vi "Util_ApproxEquals.vi"(8 "Tolerance":dbl=1e-09, 10 "Value 2":dbl, 11 "Value 1":dbl) -> (3 "ApproxEquals":bool)   [LabVIEW 2019]
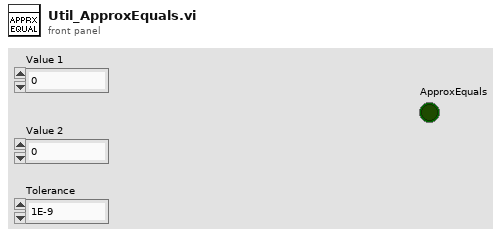
[diagram p1: front panel]
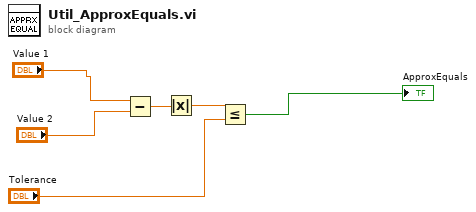
[diagram p0: block diagram]
diagram:
  n1 = Subtract(x="Value 1", y="Value 2") -> (x-y=w4:dbl)
  n2 = Absolute Value(x=w4) -> (abs(x)=w3:dbl)
  n3 = Less Or Equal?(x=w3, y="Tolerance") -> (x <= y?=→"ApproxEquals":bool)
